vi "GetActiveFieldName.vi"(1 "protobuf index":i32) -> (0 "oneof field name":string)   [LabVIEW 2019, in "xnet-grpc_client.lvlib" / "nixnet_grpc_GetPropertyResponse_property_value.lvclass"]
uses:
  nixnet_grpc_GetPropertyResponse_property_value.lvclass
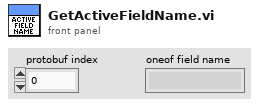
[diagram p1: front panel]
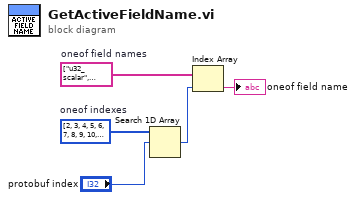
[diagram p0: block diagram]
diagram:
  w5 = string[] ["u32_scalar", "bool_scalar", "str", "u64_scalar", "i32_scalar", "f64_scalar", "string_array", "u32_array", "db_ref", "db_ref_array", "dev_ref", "dev_ref_array", "intf_ref_array", "ept_rx_filter_array"]  # oneof field names
  w4 = i32[] [2, 3, 4, 5, 6, 7, 8, 9, 10, 11, 12, 13, 14, 15]  # oneof indexes
  n1 = Search 1D Array(1D array=w4, element="protobuf index") -> (index of element=w2:i32)  [unwired: 1 in]
  n2 = Index Array(array=w5, index=w2) -> (element=→"oneof field name":string)
